vi "Mean Duration of Active Alarms.vi"(8 "error in (no error)":errorcluster, 11 "alarms in":refnum<class "NI SystemLink Alarm.lvclass">[](array[class])) -> (0 "error out":errorcluster, 1 "Average duration of active alarms (days)":dbl format="%#.2g", 2 "Average duration of active alarms (HH:MM:SS)":dbl format="%<%H:%M:%S>t", 3 "alarms out":refnum<class "NI SystemLink Alarm.lvclass">[](array[class]), 4 "Duration of active alarms (array)":dbl[](array[numeric]) format="%<%H:%M:%S>t", 5 "#of active alarms":i32)   [LabVIEW 2019, in "SystemLink Alarm KPIs.lvlib"]
uses:
  SystemLink Alarm KPIs.lvlib
  <vilib>/Skyline/Alarm/Class/NI SystemLink Alarm.lvclass
  <vilib>/Skyline/Alarm/Class/NI SystemLink Alarm.lvclass/NI SystemLink Alarm.ctl
  <vilib>/Skyline/Alarm/Class/Accessors/Read Active.vi
  <vilib>/Analysis/baseanly.llb/Mean (DBL).vi
  <vilib>/Skyline/Alarm/Class/Private/Ensure Alarm Information.vi
  <vilib>/Skyline/Alarm/Class/Accessors/Read Transitions.vi
  <vilib>/Skyline/Alarm/Library/Get Alarm Information.vi
  <vilib>/Analysis/NI_AALBase.lvlib
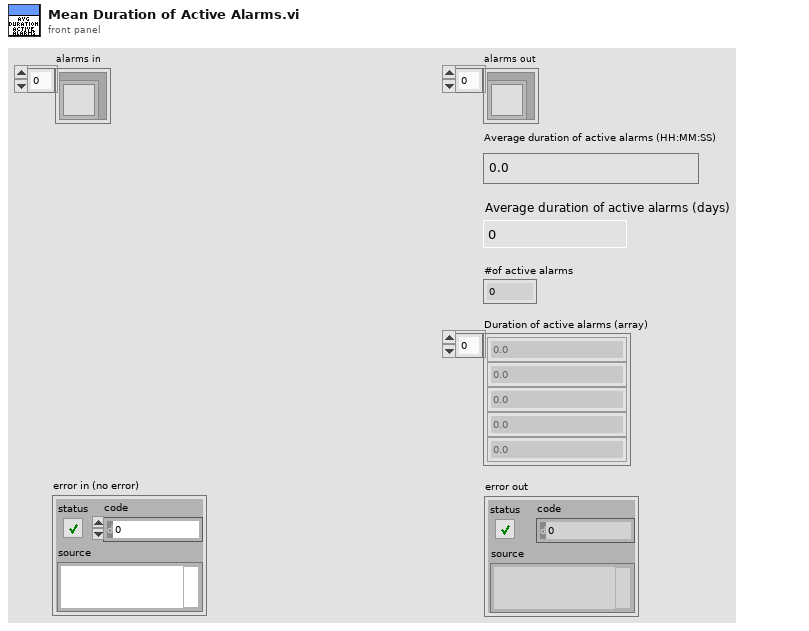
[diagram p1: front panel]
types:
  T1 = typedef "NI SystemLink Alarm Library.lvlib/Transition.ctl" = cluster{"type":T2, "severity level":T3, "condition":string, "occurred at":timestamp, "keywords":string[], "properties":T4[]}
  T2 = typedef "NI SystemLink Alarm Library.lvlib/Transition Type.ctl" = enum16{"Set", "Clear"}
  T3 = typedef "NI SystemLink Alarm Library.lvlib/Severity Level.ctl" = i32
  T4 = typedef "NI Skyline Utilities.lvlib/Property.ctl" = cluster{"key":string, "value":string}
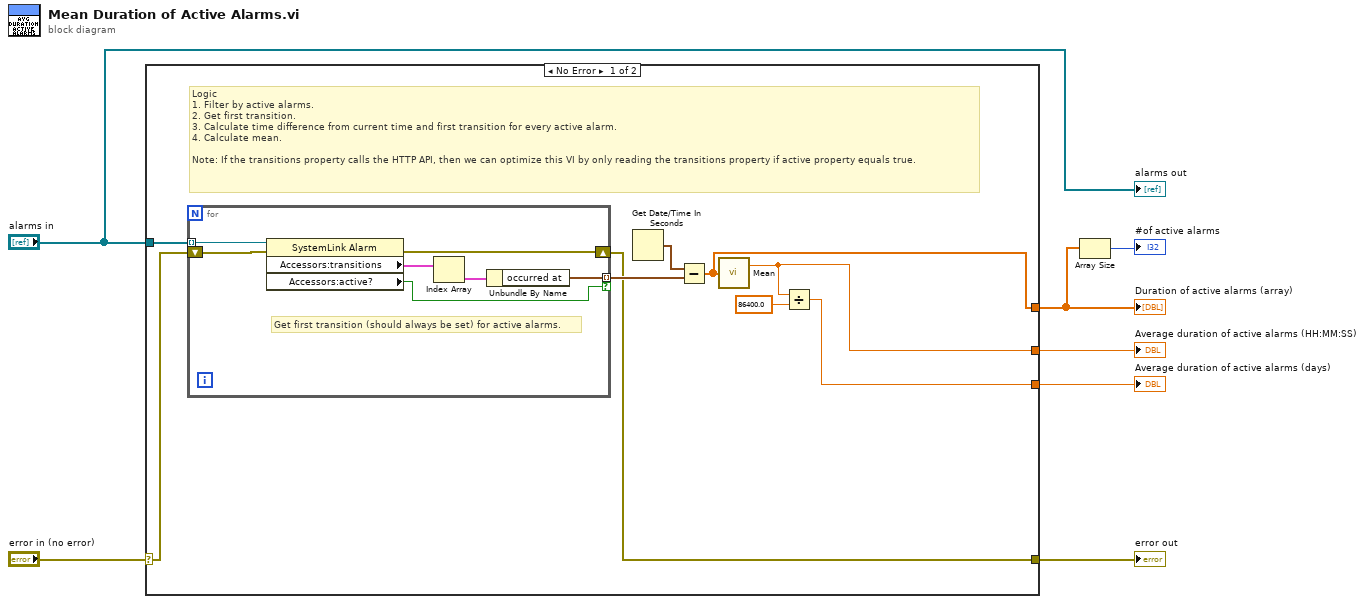
[diagram p0: block diagram]
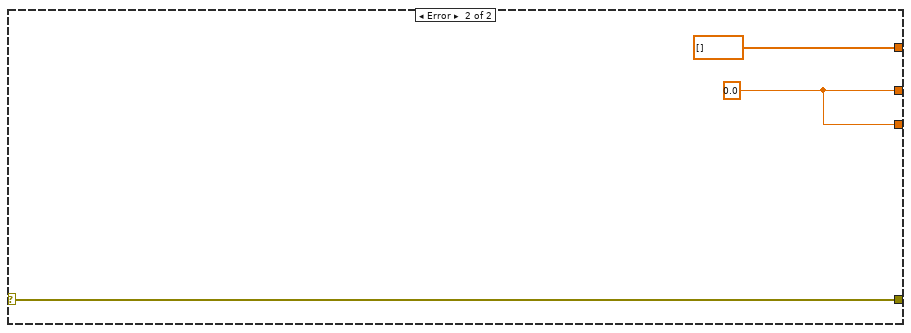
[diagram p2: hidden frame]
diagram:
  n1 = case shown="No Error" "error in (no error)" {
    selector: "error in (no error)" -> [w12 w24]
    tunnel: [w8 dbl[] []] -> w1
    tunnel: [w9 w25] -> w7
    tunnel: "alarms in" -> [w13 _]
    tunnel: [w10 w25] -> w5
    tunnel: [w11 w24] -> w3
    frame No Error {
      # "Logic\n1. Filter by active alarms.\n2. Get first transition.\n3. Calculate time difference from current time and first transition for every active alarm.\n4. Calculate mean.\n\nNote: If the transitions property calls the HTTP API, then we can optimize this VI by only reading the transitions property if active property equals true."
      n2 = for {
        tunnel: w13 -> [w23] mode=indexing
        tunnel: [w20] -> w16 mode=indexing if=w17
        shift-right: [w18] -> w11
        shift-left: w12 -> [w19]
        # "Get first transition (should always be set) for active alarms."
        n3 = property class="SystemLink Alarm"(reference=w23, error in=w19) -> (error out=w18:errorcluster, "Accessors:transitions"=w22:T1[], "Accessors:active?"=w17:bool)  [unwired: 1 out]
        n4 = Index Array(array=w22) -> (element=w21:T1)  [unwired: 1 in]
        n5 = Unbundle By Name(w21) -> ("occurred at"=w20:timestamp)
      }
      n6 = Get Date/Time In Seconds() -> (seconds since 1Jan1904=w14:timestamp)
      n7 = Subtract(x=w14, y=w16) -> (x-y=w8:dbl[])
      n8 = call-poly <vilib>:"Mean.vi"("X"=w8) -> ("mean"=w10:dbl)  [unwired: 1 out]
      n9 = Divide(x=w10, y=86400.0) -> (x/y=w9:dbl)
    }
    frame Error {
      w25 = 0.0 ("mean")
    }
  }
  "Duration of active alarms (array)" <- w1
  "Average duration of active alarms (HH:MM:SS)" <- w5
  "Average duration of active alarms (days)" <- w7
  "error out" <- w3
  n10 = Array Size(array=w1) -> (size(s)=→"#of active alarms":i32)
  "alarms out" <- "alarms in"
